vi "Text.vi"(4 "Properties":T1={"Text"={"Color"=2147483647, "Background Color"=2147483647, "Font Size (points)"=0, "Font Style"=enum."Automatic", "Rotation Angle"=nan}, "Display"={"Alpha"=nan, "Z Order"=nan}} {"Text"."Background Color" items=["Automatic"=2147483647, "Black"=0, "White"=16777215, "Red"=16711680, "Green"=2263842, "Blue"=255, "Cyan"=65535, "Magenta"=16711935, "Yellow"=16776960]; "Text"."Font Size (points)" items=["Automatic"=0, "XX-Small"=-1, "X-Small"=-2, "Small"=-3, "Medium"=-4, "Large"=-5, "X-Large"=-6, "XX-Large"=-7]; "Text"."Color" items=["Automatic"=2147483647, "Black"=0, "White"=16777215, "Red"=16711680, "Green"=2263842, "Blue"=255, "Cyan"=65535, "Magenta"=16711935, "Yellow"=16776960]}, 5 "Relative Coordinates":bool, 7 "Text":string, 8 "error in (no error)":errorcluster, 9 "Y Position":dbl, 10 "X Position":dbl, 11 "Plot ID":T7 format="%x") -> (0 "error out":errorcluster, 3 "Plot ID Out":T7 format="%x")   [LabVIEW 2013, in "Advanced Plotting Toolkit.lvlib"]
doc: "Add text to the plot."
uses:
  Advanced Plotting Toolkit.lvlib
  typedefs/PlotID.ctl
  TextProperties.ctl
  properties/Text.ctl
  typedefs/PlotColor.ctl
  properties/Text_FontSize.ctl
  properties/Text_FontStyle.ctl
  properties/Display.ctl
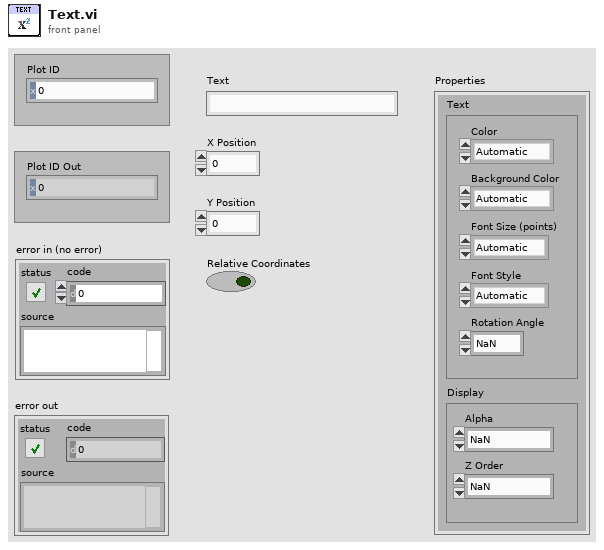
[diagram p1: front panel]
types:
  T1 = typedef "Advanced Plotting Toolkit.lvlib/TextProperties.ctl" = cluster{"Text":T2, "Display":T6}
  T2 = typedef "Advanced Plotting Toolkit.lvlib/Text.ctl" = cluster{"Color":T3, "Background Color":T3, "Font Size (points)":T4, "Font Style":T5, "Rotation Angle":dbl}
  T3 = typedef "Advanced Plotting Toolkit.lvlib/PlotColor.ctl" = u32
  T4 = typedef "Advanced Plotting Toolkit.lvlib/Text_FontSize.ctl" = i32
  T5 = typedef "Advanced Plotting Toolkit.lvlib/Text_FontStyle.ctl" = enum16{"Automatic", "Normal", "Italic", "Bold"}
  T6 = typedef "Advanced Plotting Toolkit.lvlib/Display.ctl" = cluster{"Alpha":dbl, "Z Order":dbl}
  T7 = typedef "Advanced Plotting Toolkit.lvlib/PlotID.ctl" = i32
  T8 = typedef "Advanced Plotting Toolkit.lvlib/KeyValue.ctl" = cluster{"Key":string, "Value":string}
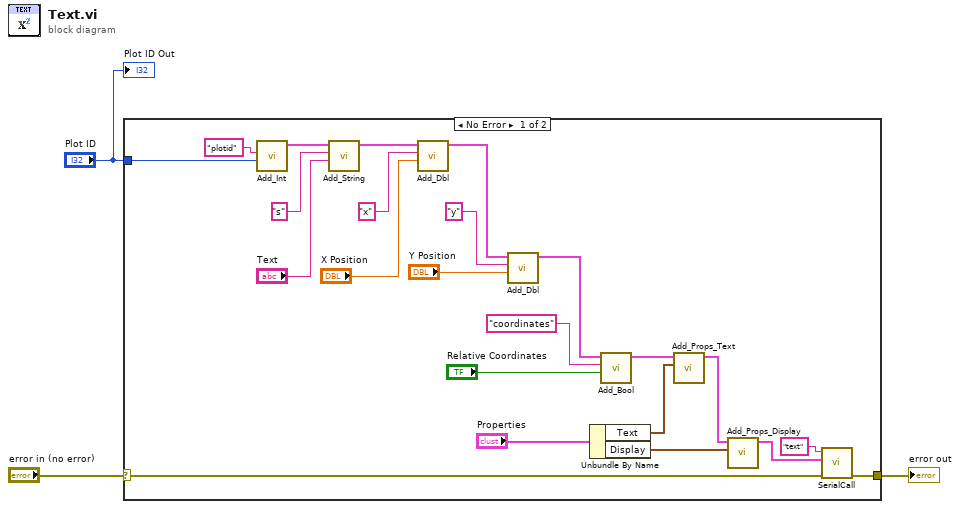
[diagram p0: block diagram]
diagram:
  n1 = case shown="No Error" "error in (no error)" {
    selector: "error in (no error)" -> [w15 w27]
    tunnel: "Plot ID" -> [w13 _]
    tunnel: [w14 w27] -> w1
    frame No Error {
      n2 = call "Add_Int.vi"("Value"=w13, "Key"="plotid") -> ("Keyword Array Out"=w16:T8[])  [unwired: 9 in]
      n3 = call "Add_String.vi"("Value"="Text", "Key"="s", "Keyword Array"=w16) -> ("Keyword Array Out"=w24:T8[])  [unwired: 8 in]
      n4 = call "Add_Dbl.vi"("Value"="X Position", "Key"="x", "Keyword Array"=w24) -> ("Keyword Array Out"=w22:T8[])  [unwired: 8 in]
      n5 = call "Add_Dbl.vi"("Value"="Y Position", "Key"="y", "Keyword Array"=w22) -> ("Keyword Array Out"=w19:T8[])  [unwired: 8 in]
      n6 = Unbundle By Name("Properties") -> ("Text"=w7:T2, "Display"=w4:T6)
      n7 = call "Add_Bool.vi"("Value"="Relative Coordinates", "Key"="coordinates", "Keyword Array"=w19) -> ("Keyword Array Out"=w9:T8[])  [unwired: 8 in]
      n8 = call "Add_Props_Text.vi"("Text Properties"=w7, "Keyword Array"=w9) -> ("Keyword Array Out"=w6:T8[])  [unwired: 9 in]
      n9 = call "Add_Props_Display.vi"("Display"=w4, "Keyword Array"=w6) -> ("Keyword Array Out"=w5:T8[])  [unwired: 9 in]
      n10 = call "SerialCall.vi"("error in (no error)"=w15, "data"=w5, "Resource"="text") -> ("error out"=w14:errorcluster)  [unwired: 7 in, 1 out]
    }
    frame Error {
    }
  }
  "error out" <- w1
  "Plot ID Out" <- "Plot ID"
